vi "Deadzone.vi"(2 "Deadzone":dbl, 3 "Input Signal":dbl) -> (0 "Output Signal":dbl, 1 "In Deadzone?":bool)   [LabVIEW 2015]
doc: "Help by FRC Team 836 - The RoboBees\n\nThis VI allows the user to define a \"Deadzone\" for whatever numerical parameter is desired. The VI will compare the\ninput signal to the user defined deadzone.\n\nIf the input is in the deadzone a \"0\" is output.\n\nIf outside the deadzone the input signal is passed through.\n\nA front panel indication is given of the comparison result."
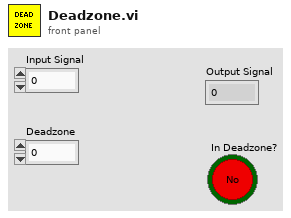
[diagram p1: front panel]
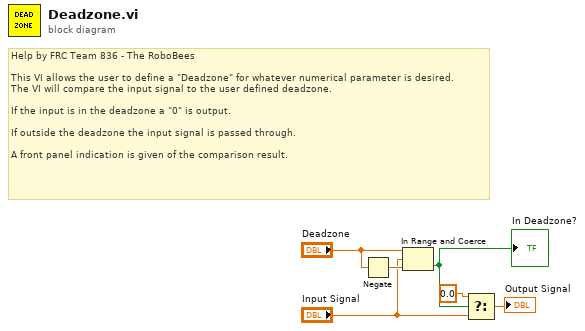
[diagram p0: block diagram]
diagram:
  # "Help by FRC Team 836 - The RoboBees\n\nThis VI allows the user to define a \"Deadzone\" for whatever numerical parameter is desired.\nThe VI will compare the input signal to the user defined deadzone.\n\nIf the input is in the deadzone a \"0\" is output.\n\nIf outside the deadzone the input signal is passed through.\n\nA front panel indication is given of the comparison result."
  n1 = Negate(x="Deadzone") -> (-x=w5:dbl)
  n2 = In Range and Coerce(upper limit="Deadzone", x="Input Signal", lower limit=w5) -> (In Range?=w4:bool)  [unwired: 1 out]
  "In Deadzone?" <- w4
  n3 = Select(t=0.0, s=w4, f="Input Signal") -> (s? t:f=→"Output Signal":dbl)
